vi "test Basic Resolution.vi"(8 "error in (no error)":errorcluster, 11 "TestCase in":refnum<class "Task Tests.lvclass">) -> (0 "error out":errorcluster, 3 "TestCase out":refnum<class "Task Tests.lvclass">)   [LabVIEW 2017, in "Task Tests.lvclass"]
uses:
  Task Tests.lvclass
  <vilib>/addons/_JKI Toolkits/VI Tester/TestCase.llb/TestCase.lvclass
  Futures/Task/Task.lvclass
  C:/Program Files (x86)/National Instruments/LabVIEW 2017/vi.lib/addons/_JKI Toolkits/VI Tester/TestCase.llb/TestCase.lvclass
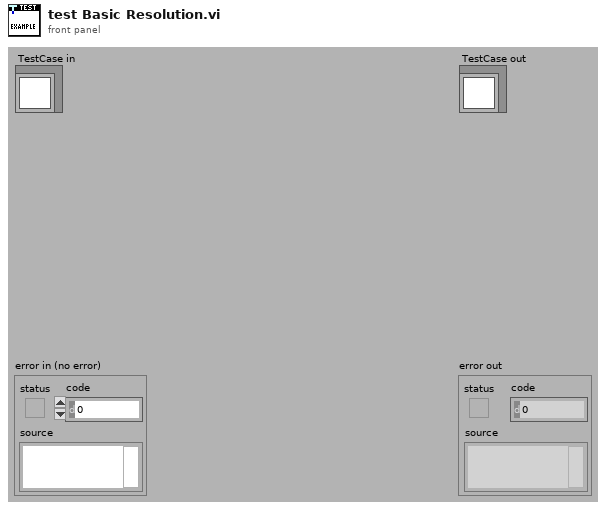
[diagram p1: front panel]
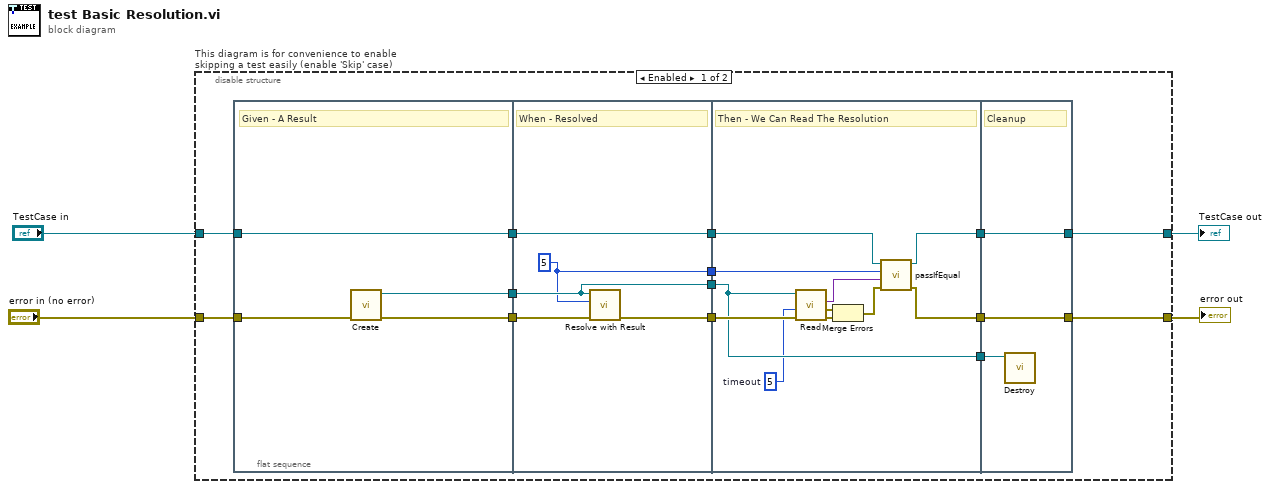
[diagram p0: block diagram]
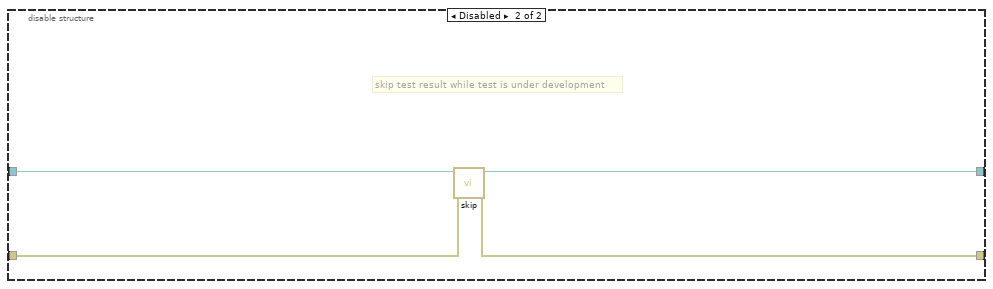
[diagram p2: hidden frame]
diagram:
  n1 = disable-structure "This diagram is for convenience to enable skipping a test easily (enable 'Skip' case)" shown="Enabled" {
    disable-tunnel: "TestCase in" -> [w12 w45]
    disable-tunnel: [w10 w43] -> w1
    disable-tunnel: [w9 w44] -> w3
    disable-tunnel: "error in (no error)" -> [w11 w42]
    frame Enabled {
      n2 = flat-sequence {
        tunnel: w11 -> [w21]
        tunnel: w12 -> [w22]
        tunnel: [w22] -> w18
        tunnel: [w20] -> w17
        tunnel: [w19] -> w8
        tunnel: [w27] -> w16
        tunnel: [w25] -> w15
        tunnel: w18 -> [w27]
        tunnel: w17 -> [w26]
        tunnel: w8 -> [w24]
        tunnel: [w24] -> w7
        tunnel: [w23] -> w6
        tunnel: [w37] -> w14
        tunnel: [w36] -> w13
        tunnel: w16 -> [w38]
        tunnel: w15 -> [w35]
        tunnel: w7 -> [w29]
        tunnel: w6 -> [w30]
        tunnel: [w29] -> w5
        tunnel: [w40] -> w9
        tunnel: [w41] -> w10
        tunnel: w14 -> [w41]
        tunnel: w13 -> [w40]
        tunnel: w5 -> [w39]
        frame #0 {
          # "Given - A Result"
          n3 = call "Create.vi"("error in (no error)"=w21) -> ("error out"=w20:errorcluster, "Result out"=w19:refnum<class "Task.lvclass">)  [unwired: 9 in]
        }
        frame #1 {
          w23 = 5
          # "When - Resolved"
          n4 = call "Resolve with Result.vi"("error in (no error)"=w26, "Result"=w23, "Result in"=w24) -> ("error out"=w25:errorcluster)  [unwired: 8 in]
        }
        frame #2 {
          w28 = 5  # timeout
          # "Then - We Can Read The Resolution"
          n5 = call "Read.vi"("error in (no error)"=w35, "timeout in ms (60 sec)"=w28, "Result in"=w29) -> ("error out"=w34:errorcluster, "result error"=w32:errorcluster, "Result value"=w31:variant)  [unwired: 4 in, 2 out]
          n6 = Merge Errors(w32, w34) -> (w33:errorcluster)
          n7 = call-dynamic "passIfEqual.vi"("error in (no error)"=w33, "y"=w31, "x"=w30, "TestCase in"=w38) -> ("error out"=w36:errorcluster, "TestCase out"=w37:refnum<class "Task Tests.lvclass">)  [unwired: 6 in]
        }
        frame #3 {
          # "Cleanup"
          n8 = call "Destroy.vi"("Result in"=w39) -> ()  [unwired: 10 in, 1 out]
        }
      }
    }
    frame Disabled {
      # "skip test result while test is under development"
      n9 = call <vilib>:"skip.vi"("error in (no error)"=w42, "TestCase in"=w45) -> ("error out"=w44:errorcluster, "TestCase out"=w43:refnum<class "Task Tests.lvclass">)  [unwired: 8 in]
    }
  }
  "error out" <- w3
  "TestCase out" <- w1
